vi "tip_cal_objective_fun.vi"(3 "output control":T1, 4 "data":T2, 5 "X":dbl[](array[numeric])) -> (0 "error out":errorcluster, 1 "gradient":dbl[](array[numeric]), 2 "f(X)":dbl)   [LabVIEW 2013]
doc: "This template is the starting point for creating an objectivel function to be passed to the Unconstrained Optimization.vi."
uses:
  <vilib>/gmath/NumericalOptimization/objective function data.ctl
  <vilib>/gmath/NI_Gmath.lvlib
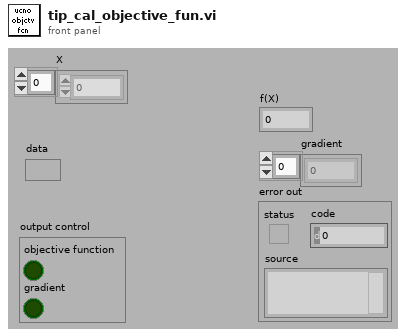
[diagram p1: front panel]
types:
  T1 = cluster{"objective function":bool, "gradient":bool}
  T2 = typedef "NI_Gmath.lvlib/objective function data.ctl" = variant
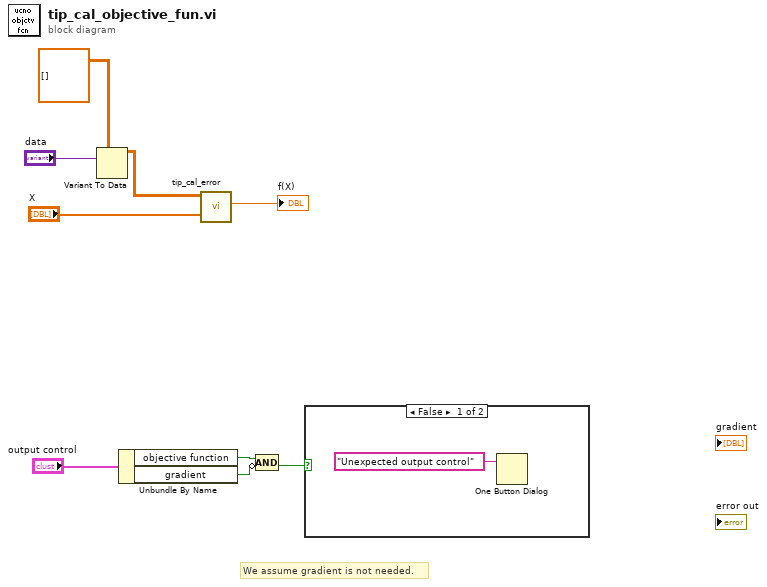
[diagram p0: block diagram]
diagram:
  # "We assume gradient is not needed."
  n1 = Variant To Data(type=dbl[][][] [] ("Calibration point pose"), Variant="data") -> (data=w2:dbl[][][])  [unwired: 1 in, 1 out]
  n2 = Unbundle By Name("output control") -> ("objective function"=w6:bool, "gradient"=w5:bool)
  n3 = call "tip_cal_error.vi"("X"="X", "Calibration point pose"=w2) -> ("f(X)"=→"f(X)":dbl)  [unwired: 2 in, 7 out]
  n4 = Compound Arithmetic op=AND(w6, invert w5) -> (w4:bool)
  n5 = case shown="False" w4 {
    frame False {
      n6 = One Button Dialog(message="Unexpected output control") -> ()  [unwired: 2 out]
    }
    frame True {
    }
  }
